vi "READ DUBAS DATALOG.vi"(7 "STATES":T1=enum."CLOSE", 8 "error in (no error)":errorcluster, 11 "DUBAS DATA IN":string[](array[string])) -> (0 "error out":errorcluster, 3 "DUBAS DATA OUT":string[](array[string]))   [LabVIEW 2018]
uses:
  Controls/DUBAS DTALOG FGV STATES.ctl
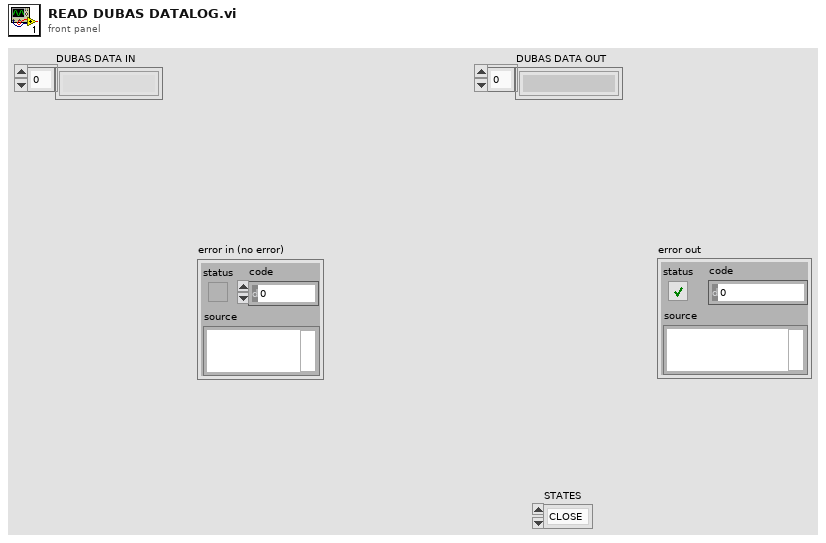
[diagram p1: front panel]
types:
  T1 = typedef "DUBAS DTALOG FGV STATES.ctl" = enum16{"OPEN REF", "READ DATA", "WRITE DATA", "CLOSE"}
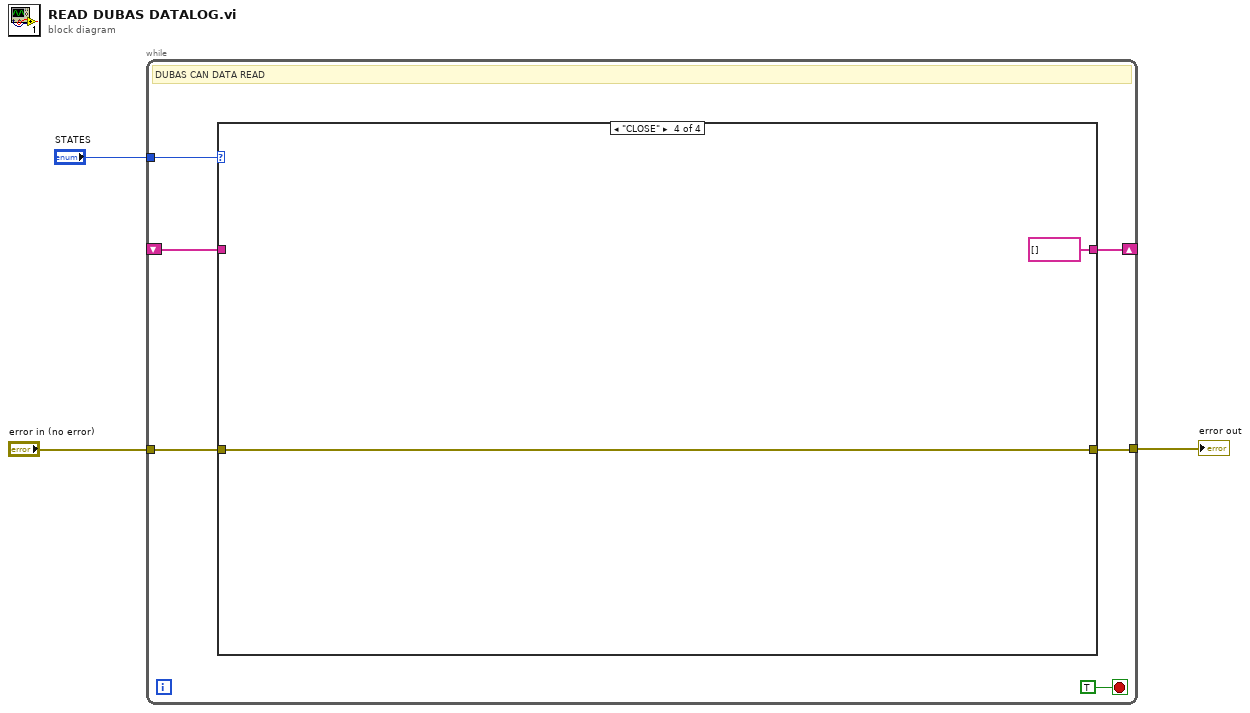
[diagram p0: block diagram]
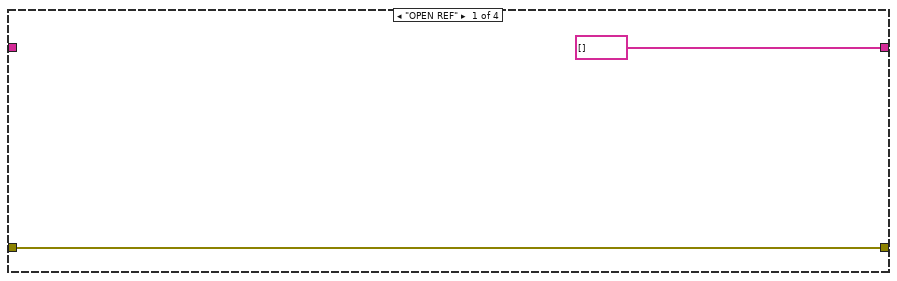
[diagram p2: hidden frame]
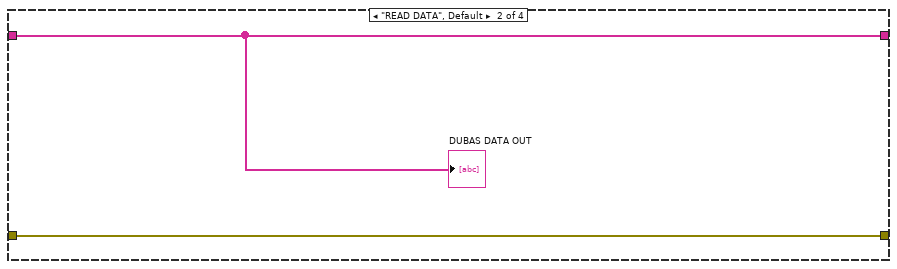
[diagram p3: hidden frame]
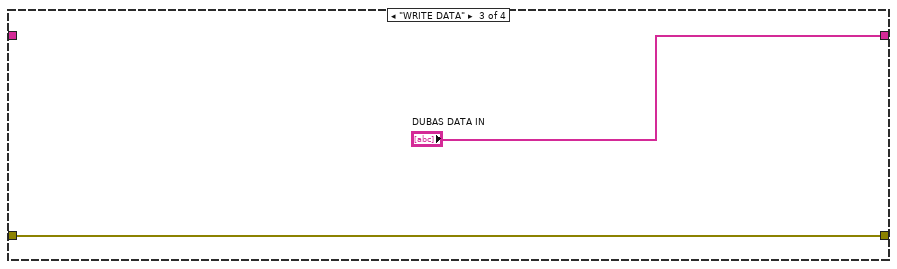
[diagram p4: hidden frame]
diagram:
  n1 = while {
    tunnel: "STATES" -> [w8]
    tunnel: "error in (no error)" -> [w7]
    tunnel: [w6] -> w1
    shift-right: [w5] -> _
    shift-left: _ -> [w4]
    stop <- TRUE stop-if-true
    # "DUBAS CAN DATA READ"
    n2 = case shown="\"CLOSE\"" w8 {
      tunnel: w7 -> [w10 w13 w14 w17]
      tunnel: [w10 w13 w14 w17] -> w6
      tunnel: [string[] [] w12 "DUBAS DATA IN" string[] [] ("DUBAS DATA IN")] -> w5
      tunnel: w4 -> [_ w12 _ _]
      frame "OPEN REF" {
      }
      frame "READ DATA", Default {
        "DUBAS DATA OUT" <- w12
      }
      frame "WRITE DATA" {
      }
      frame "CLOSE" {
      }
    }
  }
  "error out" <- w1
